vi "Write Sensitivity.vi"(8 "error in (no error)":errorcluster, 10 "Sensitivity":dbl, 11 "Sensor DAO Class in":refnum<class "Sensor DAO Class.lvclass">) -> (0 "error out":errorcluster, 3 "Sensor DAO Class out":refnum<class "Sensor DAO Class.lvclass">)   [LabVIEW 2013, in "Sensor DAO Class.lvclass"]
uses:
  Sensor DAO Class.lvclass
  Sensor DAO Class.lvclass/Sensor DAO Class.ctl
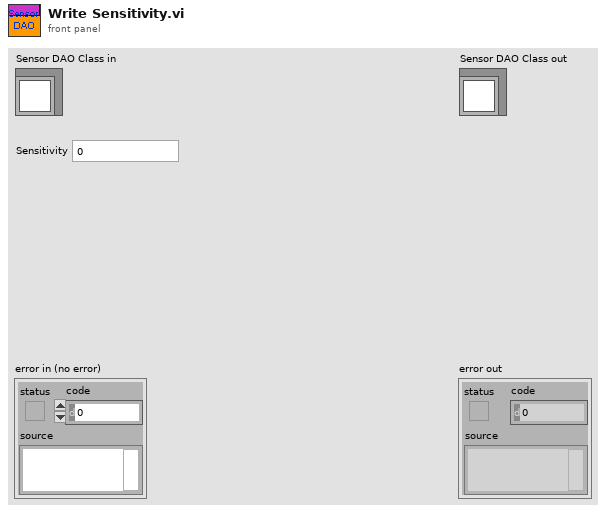
[diagram p1: front panel]
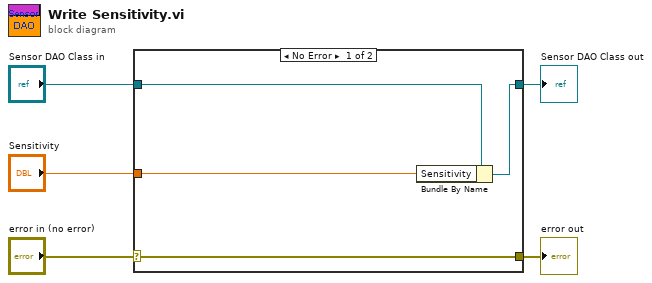
[diagram p0: block diagram]
diagram:
  n1 = case shown="No Error" "error in (no error)" {
    selector: "error in (no error)" -> [w9 w10]
    tunnel: [w9 w10] -> w4
    tunnel: [w7 w11] -> w2
    tunnel: "Sensor DAO Class in" -> [w8 w11]
    tunnel: "Sensitivity" -> [w6 _]
    frame No Error {
      n2 = Bundle By Name(cluster=w8, "Sensitivity"=w6) -> (w7:refnum<class "Sensor DAO Class.lvclass">)
    }
    frame Error {
    }
  }
  "error out" <- w4
  "Sensor DAO Class out" <- w2
